vi "Get Splitter Details.vi"(6 "Splitter Width/Height":dbl=4.0 format="%#_13g", 8 "error in (no error)":errorcluster, 9 "Offset":T1, 10 "Scale Factor":dbl, 11 "Splitters[]":refnum<vi>[](array[refnum])) -> (0 "error out":errorcluster, 3 "Splitter Details":T2[](array[typedef]))   [LabVIEW 2018]
uses:
  <resource>/dialog/QuickDrop/plugins/PaneRelief/Typedefs/Splitter Details--Cluster.ctl
  <resource>/dialog/QuickDrop/plugins/PaneRelief/Typedefs/Point--Cluster.ctl
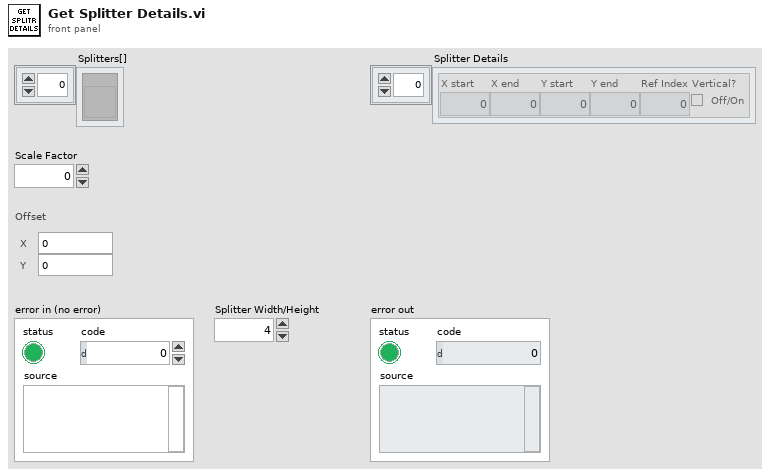
[diagram p1: front panel]
types:
  T1 = typedef "Point--Cluster.ctl" = cluster{"Horizontal":i32, "Vertical":i32}
  T2 = typedef "Splitter Details--Cluster.ctl" = cluster{"X start":i32, "X end":i32, "Y start":i32, "Y end":i32, "Ref Index":i32, "Vertical?":bool}
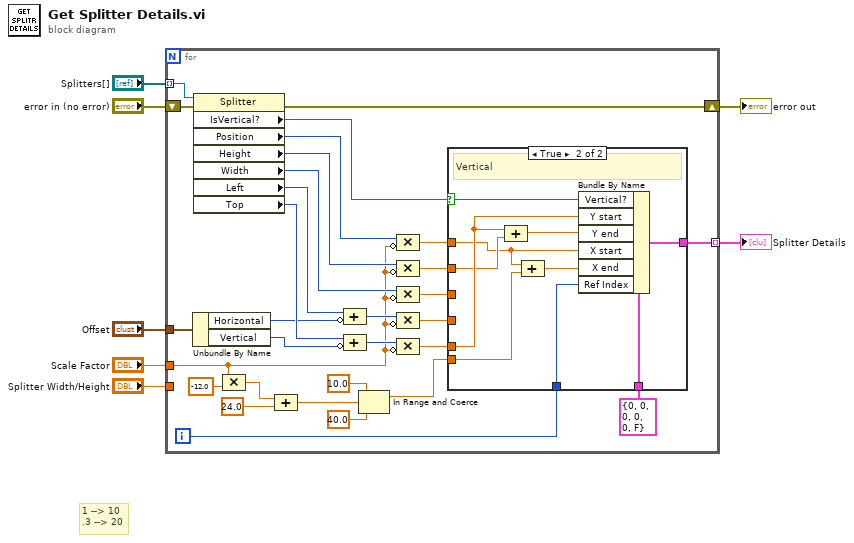
[diagram p0: block diagram]
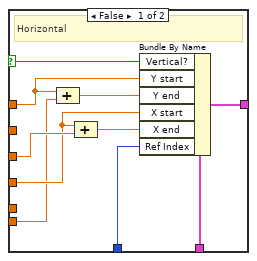
[diagram p2: hidden frame]
diagram:
  # "1 --> 10\n.3 --> 20"
  n1 = for {
    tunnel: "Splitters[]" -> [w37] mode=indexing
    tunnel: [w34] -> w6 mode=indexing
    tunnel: "Splitter Width/Height" -> [_]
    tunnel: "Scale Factor" -> [w13]
    shift-right: [w23] -> w2
    shift-left: "error in (no error)" -> [w24]
    tunnel: "Offset" -> [w20]
    i -> [w22]
    n2 = Unbundle By Name(w20) -> ("Horizontal"=w16:i32, "Vertical"=w19:i32)
    n3 = property class="Splitter"(reference=w37, error in=w24) -> (error out=w23:errorcluster, "IsVertical?"=w36:bool, "Position"=w33:i32, "Height"=w26:u32, "Width"=w29:u32, "Left"=w18:i32, "Top"=w21:i32)  [unwired: 1 out]
    n4 = Compound Arithmetic op=MULTIPLY(w13, -12.0 ("value")) -> (w11:dbl)
    n5 = Compound Arithmetic op=unknown(w11, 24.0 ("value")) -> (w9:dbl)
    n6 = Compound Arithmetic op=ADD(w18, invert w16) -> (w17:i32)
    n7 = Compound Arithmetic op=ADD(w21, invert w19) -> (w25:i32)
    n8 = In Range and Coerce(upper limit=10.0, x=w9, lower limit=40.0 ("upper limit")) -> (coerced(x)=w8:dbl)  [unwired: 1 out]
    n9 = Compound Arithmetic op=MULTIPLY(w33, invert w13) -> (w30:dbl)
    n10 = Compound Arithmetic op=MULTIPLY(w26, invert w13) -> (w31:dbl)
    n11 = Compound Arithmetic op=MULTIPLY(w29, invert w13) -> (w32:dbl)
    n12 = Compound Arithmetic op=MULTIPLY(w17, invert w13) -> (w28:dbl)
    n13 = Compound Arithmetic op=MULTIPLY(w25, invert w13) -> (w27:dbl)
    n14 = case shown="True" w36 {
      selector: w36 -> [w39 w49]
      tunnel: T2 {"X start"=0, "X end"=0, "Y start"=0, "Y end"=0, "Ref Index"=0, "Vertical?"=FALSE} -> [w38 w48]
      tunnel: w30 -> [w43 w53]
      tunnel: w28 -> [w46 _]
      tunnel: w31 -> [_ w54]
      tunnel: w32 -> [w47 _]
      tunnel: w27 -> [_ w56]
      tunnel: [w44 w55] -> w34
      tunnel: w8 -> [w41 w51]
      tunnel: w22 -> [w40 w50]
      frame False {
        # "Horizontal"
        n15 = Compound Arithmetic op=ADD(w43, w41) -> (w42:dbl)
        n16 = Compound Arithmetic op=ADD(w46, w47) -> (w45:dbl)
        n17 = Bundle By Name(cluster=w38, "Vertical?"=w39, "Y start"=w43, "Y end"=w42, "X start"=w46, "X end"=w45, "Ref Index"=w40) -> (w44:T2)
      }
      frame True {
        # "Vertical"
        n18 = Compound Arithmetic op=ADD(w56, w54) -> (w57:dbl)
        n19 = Compound Arithmetic op=ADD(w53, w51) -> (w52:dbl)
        n20 = Bundle By Name(cluster=w48, "Vertical?"=w49, "Y start"=w56, "Y end"=w57, "X start"=w53, "X end"=w52, "Ref Index"=w50) -> (w55:T2)
      }
    }
  }
  "Splitter Details" <- w6
  "error out" <- w2
